vi "Teleop.vi"(10 "Match Info":T1={"Autonomous Elapsed Seconds"=0.0, "TeleOp Elapsed Seconds"=0.0, "Disabled Elapsed Seconds"=0.0, "Visited Autonomous"=FALSE, "Visited TeleOp"=FALSE, "Visited Disabled"=FALSE, "Autonomous Settings"={"Autonomous Style"=enum."Independent", "VI Refnum"=refnum}}, 11 "Call Context":T2) -> ()   [LabVIEW 2013]
doc: "This VI is called for each TeleOp packet received from the DS where the robot is not disabled. It is often used to read from the joysticks and update I/O or to update setpoints for timed control loops. It should complete and return within 20 milliseconds or it may miss DS packets."
uses:
  <vilib>/Rock Robotics/WPI/DriverStation/WPI_DriverStationDerivedRobotMode.ctl
  <vilib>/Rock Robotics/WPI/DriverStation/WPI_DriverStationMatch Info.ctl
  <vilib>/Rock Robotics/WPI/Solenoid/WPI_SolenoidValue.ctl
  <vilib>/Rock Robotics/WPI/Ultrasonic/WPI_UltrasonicRangeUnits.ctl
  Robot Global Data.vi
  <vilib>/Rock Robotics/WPI/Solenoid/WPI_SolenoidGetEnum.vi
  <vilib>/Rock Robotics/Network Tables/SD Read Number.vi
  <vilib>/Rock Robotics/WPI/Joystick/WPI_JoystickGetSetRefNum.vi
  <vilib>/Rock Robotics/WPI/Solenoid/WPI_SolenoidSetEnum.vi
  <vilib>/Rock Robotics/WPI/RobotDrive/WPI_RobotDriveGetSetRefNum.vi
panel:
  out "Waveform Chart":dbl(graph)
  in  "Fish Tester":dbl
  out "Sensor Time":dbl
  out "Ultrasonic Distance":dbl
  out "Mechanism Moving Up":bool
  out "Mechanism Moving Down":bool
  out "Time Since Button Pressed":dbl
  in  "Manual Override Activated":bool
  in  "Button 8 Pressed":bool
  out "Button 3":bool
  out "Button 2":bool
  out "Button 1":bool
  in  "Button 3 Pressed":bool
  in  "Button 2 Pressed":bool
  in  "Firing Pin Forward":bool
  in  "Mechanism Piston Forward":bool
  in  "Tick Taken":bool
  out "Time at Gather":dbl
  out "Time After Firing":dbl
  in  "Mechanism Status":string
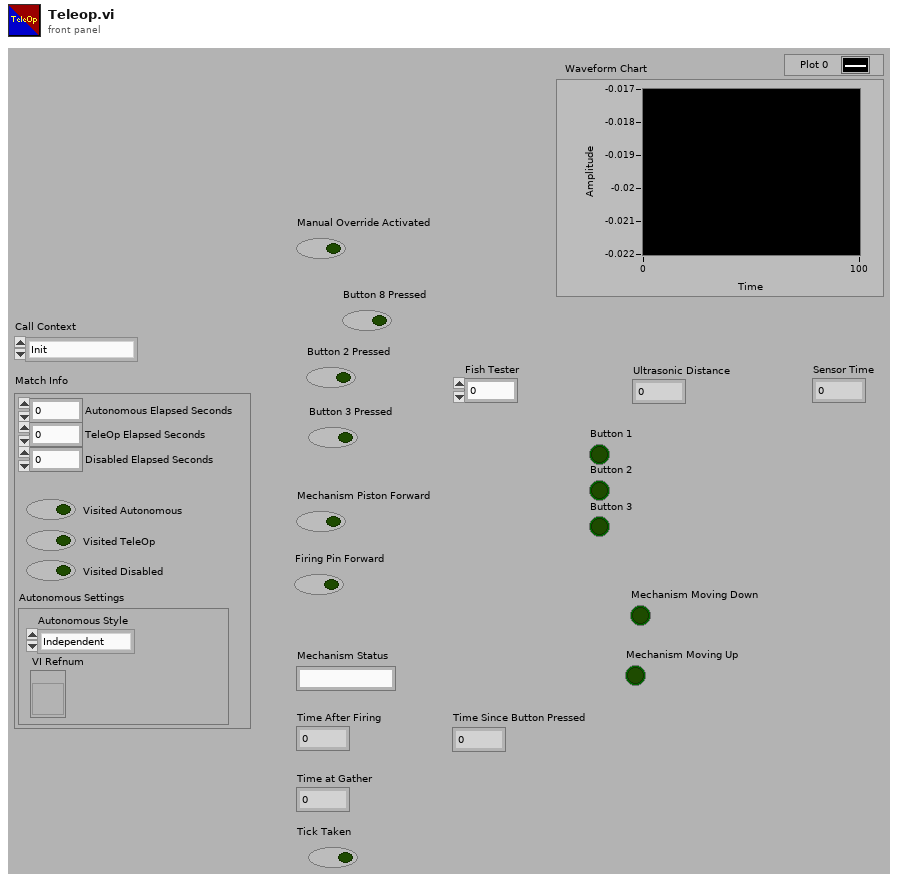
[diagram p1: front panel]
types:
  T1 = typedef "WPI_DriverStationMatch Info.ctl" = cluster{"Autonomous Elapsed Seconds":dbl, "TeleOp Elapsed Seconds":dbl, "Disabled Elapsed Seconds":dbl, "Visited Autonomous":bool, "Visited TeleOp":bool, "Visited Disabled":bool, "Autonomous Settings":cluster{"Autonomous Style":enum16{"Iterative", "Independent"}, "VI Refnum":refnum<vi>}}
  T2 = typedef "WPI_DriverStationDerivedRobotMode.ctl" = enum16{"Init", "Execute", "Stop"}
  T3 = typedef "WPI_SolenoidValue.ctl" = enum16{"Off", "On", "Forward", "Reverse"}
  T4 = typedef "WPI_JoystickDevRef.ctl" = cluster{"Device":T5}
  T5 = typedef "WPI_JoystickDeviceEnum.ctl" = enum16{"USB 1", "USB 2", "USB 3", "USB 4", "Kinect 1", "Kinect 2"}
  T6 = typedef "WPI_JoystickButtonState.ctl" = cluster{"Button 1":bool, "Button 2":bool, "Button 3":bool, "Button 4":bool, "Button 5":bool, "Button 6":bool, "Button 7":bool, "Button 8":bool, "Button 9":bool, "Button 10":bool, "Button 11":bool, "Button 12":bool}
  T7 = cluster{"axis 1 (x)":dbl, "axis 2 (y)":dbl, "axis 3 (throttle)":dbl, "axis 4":dbl, "axis 5":dbl, "axis 6":dbl}
  T8 = typedef "WPI_RobotDriveDevRef.ctl" = cluster{"DevStatus":errorcluster, "Motors[]":T9[], "Square Inputs":bool, "Max Output":dbl, "Isochronous":bool}
  T9 = typedef "WPI_MotorControlDeviceRef.ctl" = cluster{"DeviceStatus":errorcluster, "Type":enum16{"PWM", "CAN"}, "PWM":cluster{"Digital Module":T10, "PWM Channel":T11, "DeadBand":T12}, "CAN":cluster{"Device Number":u8, "Control Mode":T13, "Semaphore":T14, "Max Vout":dbl}, "Invert":bool, "TransformRef":T15, "InvTransformRef":T15}
  T10 = typedef "FPGA_TypedefDigitalModule.ctl" = enum16{"Digital Module 1", "Digital Module 2"}
  T11 = typedef "FPGA_DIOPWMChannel.ctl" = enum8{"PWM 1", "PWM 2", "PWM 3", "PWM 4", "PWM 5", "PWM 6", "PWM 7", "PWM 8", "PWM 9", "PWM 10", "Invalid"}
  T12 = typedef "WPI_PWMDeadband.ctl" = cluster{"Name":string, "maxPositivePwm":i32, "minPositivePwm":i32, "centerPwm":i32, "maxNegativePwm":i32, "minNegativePwm":i32, "angularRange":u16}
  T13 = typedef "WPI_CANJaguar_ControlMode.ctl" = enum8{"Percent VBus", "Current", "Speed", "Position", "Voltage"}
  T14 = typedef "Semaphore RefNum" = refnum<k1>
  T15 = typedef "WPI_PWMTransform_ConPane.ctl" = refnum<vi>
  T16 = typedef "WPI_SolenoidDevRef.ctl" = cluster{"DevStatus":errorcluster, "Solenoid Module":T17, "Forward Solenoid Channel":T18, "Reverse Solenoid Channel":T18}
  T17 = typedef "FPGA_TypedefSolenoidModule.ctl" = enum16{"Solenoid Module 1", "Solenoid Module 2"}
  T18 = typedef "WPI_SolenoidChannel.ctl" = enum8{"Solenoid 1", "Solenoid 2", "Solenoid 3", "Solenoid 4", "Solenoid 5", "Solenoid 6", "Solenoid 7", "Solenoid 8", "Invalid"}
  T19 = typedef "WPI_DigitalInputDevRef.ctl" = cluster{"DevStatus":errorcluster, "DIO Channel":T20, "Digital Module":T10}
  T20 = typedef "FPGA_DIOChannel.ctl" = enum8{"DIO 1", "DIO 2", "DIO 3", "DIO 4", "DIO 5", "DIO 6", "DIO 7", "DIO 8", "DIO 9", "DIO 10", "DIO 11", "DIO 12", "DIO 13", "DIO 14", "Invalid"}
  T21 = typedef "WPI_UltrasonicRangeUnits.ctl" = enum16{"inches", "mm"}
  T22 = typedef "WPI_UltrasonicDeviceRef.ctl" = cluster{"DevStatus":errorcluster, "Ping Digital Module":T10, "Echo Digital Module":T10, "Ping Channel":T20, "Echo Channel":T20, "CntIndex":T23}
  T23 = typedef "FPGA_CounterCtrSystemIndex.ctl" = enum8{"Ctr 0", "Ctr 1", "Ctr 2", "Ctr 3", "Ctr 4", "Ctr 5", "Ctr 6", "Ctr 7", "Invalid"}
  T24 = typedef "WPI_ServoDeviceRef.ctl" = cluster{"DeviceStatus":errorcluster, "Digital Module":T10, "PWM Channel":T11, "DeadBand":T12}
  T25 = typedef "WPI_AnalogChannelDevRef.ctl" = cluster{"DevStatus":errorcluster, "Analog Module":T26, "Analog Channel":T27}
  T26 = typedef "FPGA_TypedefAnalogModule.ctl" = enum16{"Analog Module 1", "Analog Module 2"}
  T27 = typedef "FPGA_AIChannel.ctl" = enum8{"AI 1", "AI 2", "AI 3", "AI 4", "AI 5", "AI 6", "AI 7", "AI 8", "Invalid"}
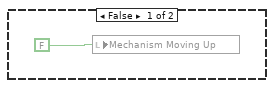
[diagram p2: hidden frame]
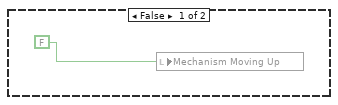
[diagram p3: hidden frame]
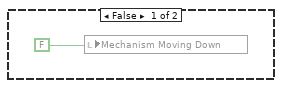
[diagram p4: hidden frame]
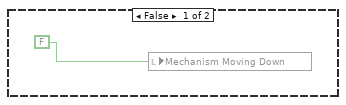
[diagram p5: hidden frame]
diagram:
  (unwired) "This code sets the toggle rate used by the Periodic Tasks VI.  For teleop mode we flash the USER1 LED on the cRIO at a fast rate.  Look at the Periodic Tasks VI to see how this global value is used."
  (unwired) "This VI is called each time a TeleOp DS packet is received.  Use it to respond to new joystick or Driver Station values.\n\nCommon tasks include reading the joysticks and updating motors, and updating setpoints for periodic loops.\n\nYou can open I/O on the FIRST Call, or in the Begin.vi."
  # "If no buttons pressed - 0\nIf left pressed = 7\nIf right pressed = -7\nIf both = 0"
  # "These are examples of reading dashboard variables."
  # "Publish the Robot Drive Motor\nvalues to the dashboard"
  # "Publish the joystick data the\nrobot sees to the dashboard"
  # "Each time we enter, report that\nwe are running teleop"
  # "Use to differentiate between\nFirst, Last, and Intermediate calls"
  # "This can help determine what has\nbeen run and for how long"
  # "Read Joystick X and Y values and update motor values"
  n1 = Unbundle By Name("Match Info") -> ()  [unwired: 1 out]
  n2 = local read "Time After Firing"() -> (w69:dbl)
  n3 = local read "Mechanism Status"() -> (w74:string)
  n4 = local write "Mechanism Piston Forward"(FALSE) -> ()
  n5 = local write "Firing Pin Forward"(FALSE) -> ()
  n6 = call <vilib>:"WPI_DriverStationReport Robot Code State.vi"("TeleOp"=TRUE ("Autonomous")) -> ()  [unwired: 10 in, 1 out]
  n7 = global write "Robot Global Data.vi" "LED toggle rate (ms)"(u32 100 ("LED ms toggle rate")) -> ()
  n8 = local read "Mechanism Status"() -> (w71:string)
  n9 = call <vilib>:"WPI_JoystickRefNum Registry Get.vi"("refnum name"="Joystick 1") -> ("JoystickDevRef"=w58:T4)  [unwired: 1 in, 9 out]
  n10 = call <vilib>:"WPI_JoystickRefNum Registry Get.vi"("refnum name"="Joystick 1") -> ("JoystickDevRef"=w76:T4)  [unwired: 1 in, 9 out]
  n11 = call <vilib>:"WPI_JoystickGet.vi"("JoystickDevRef"=w58) -> ("Buttons"=w57:T6)  [unwired: 1 in, 5 out]
  n12 = call <vilib>:"WPI_JoystickGet.vi"("JoystickDevRef"=w76) -> ("Buttons"=w75:T6, "Axes"=w55:T7)  [unwired: 1 in, 4 out]
  n13 = Tick Count (ms)() -> (millisecond timer value=w66:u32)
  n14 = call <vilib>:"WPI_RobotDriveRefNum Registry Get.vi"("refnum name"="Left and Right Motors") -> ("RobotDriveDevRef"=w90:T8)  [unwired: 1 in, 9 out]
  n15 = Unbundle By Name(w57) -> ("Button 8"=w56:bool)
  n16 = Unbundle By Name(w55) -> ()  [unwired: 1 out]
  n17 = call <vilib>:"WPI_SolenoidRefNum Registry Get.vi"("refnum name"="Firing Pin Solenoid") -> ("SolenoidDevRef"=w38:T16)  [unwired: 9 in, 1 out]
  n18 = call <vilib>:"SD Read Boolean.vi"("Name"="Manual Mechanism Override") -> ("Boolean"=w41:bool)  [unwired: 8 in, 2 out]
  n19 = call <vilib>:"WPI_SolenoidRefNum Registry Get.vi"("refnum name"="Mechanism Solenoid") -> ("SolenoidDevRef"=w32:T16)  [unwired: 9 in, 1 out]
  n20 = Subtract(x=w66, y=w69) -> (x-y=w68:dbl)
  n21 = Equal?(x=w74, y="Firing") -> (x = y?=w72:bool)
  n22 = case shown="True" w72 {
    frame False {
    }
    frame True {
      n23 = Tick Count (ms)() -> (millisecond timer value=w94:u32)
      n24 = local write "Firing Pin Forward"(FALSE) -> ()
      n25 = local write "Time After Firing"(w94) -> ()
      n26 = local write "Mechanism Status"("Resetting") -> ()
      n27 = call <vilib>:"WPI_SolenoidRefNum Registry Get.vi"("refnum name"="Firing Pin Solenoid") -> ("SolenoidDevRef"=w97:T16)  [unwired: 9 in, 1 out]
      n28 = call-poly <vilib>:"WPI_SolenoidSet.vi"("Value"=WPI_SolenoidValue."Reverse", "SolenoidDevRef"=w97) -> ()  [unwired: 8 in, 2 out]
    }
  }
  n29 = case shown="True" w41 {
    tunnel: w38 -> [_ w114]
    tunnel: w32 -> [_ w113]
    frame False {
    }
    frame True {
      n30 = call <vilib>:"SD Read Boolean.vi"("Name"="Firing Pin Piston Extended") -> ("Boolean"=w104:bool)  [unwired: 8 in, 2 out]
      n31 = call <vilib>:"SD Read Boolean.vi"("Name"="Mechanism Piston Extended") -> ("Boolean"=w111:bool)  [unwired: 8 in, 2 out]
      n32 = Equal?(x=w104, y=TRUE) -> (x = y?=w102:bool)
      n33 = Equal?(x=w111, y=TRUE) -> (x = y?=w109:bool)
      n34 = Select(t=WPI_SolenoidValue."Forward" ("Value"), s=w102, f=WPI_SolenoidValue."Reverse") -> (s? t:f=w99:T3)
      n35 = Select(t=WPI_SolenoidValue."Forward" ("Value"), s=w109, f=WPI_SolenoidValue."Reverse") -> (s? t:f=w106:T3)
      n36 = call-poly <vilib>:"WPI_SolenoidSet.vi"("Value"=w99, "SolenoidDevRef"=w114) -> ()  [unwired: 8 in, 2 out]
      n37 = call-poly <vilib>:"WPI_SolenoidSet.vi"("Value"=w106, "SolenoidDevRef"=w113) -> ()  [unwired: 8 in, 2 out]
    }
  }
  n38 = Unbundle By Name(w75) -> ("Button 1"=w60:bool, "Button 2"=w28:bool, "Button 3"=w27:bool, "Button 5"=w46:bool, "Button 6"=w47:bool)
  "Button 1" <- w60
  "Button 3" <- w27
  "Button 2" <- w28
  n39 = disable-structure shown="Disabled" {
    disable-tunnel: w28 -> [w116 _]
    disable-tunnel: w27 -> [w115 _]
    frame Disabled {
      n40 = case shown="True" w116 {
        frame False {
          n41 = local write "Mechanism Moving Down"(FALSE) -> ()
        }
        frame True {
          n42 = call <vilib>:"WPI_DigitalInputRefNum Registry Get.vi"("refnum name"="Bottom Limit Switch") -> ("DigitalInputDevRef"=w129:T19)  [unwired: 9 in, 1 out]
          n43 = call <vilib>:"WPI_DigitalInputGetValue.vi"("DigitalInputDevRef"=w129) -> ("Value"=w127:bool)  [unwired: 8 in, 2 out]
          n44 = case shown="True" w127 {
            frame False {
              n45 = local write "Mechanism Moving Down"(FALSE) -> ()
            }
            frame True {
              n46 = call <vilib>:"WPI_MotorControlRefNum Registry Get.vi"("refnum name"="Mechanism Motor 1") -> ("MotorControlDevRef"=w133:T9)  [unwired: 9 in, 1 out]
              n47 = call <vilib>:"WPI_MotorControlSetOutput.vi"("Output"=-0.1, "MotorControlDevRef"=w133) -> ()  [unwired: 7 in, 3 out]
              n48 = local write "Mechanism Moving Down"(TRUE) -> ()
            }
          }
        }
      }
      n49 = case shown="True" w115 {
        frame False {
          n50 = local write "Mechanism Moving Up"(FALSE) -> ()
        }
        frame True {
          n51 = call <vilib>:"WPI_DigitalInputRefNum Registry Get.vi"("refnum name"="Top Limit Switch") -> ("DigitalInputDevRef"=w120:T19)  [unwired: 9 in, 1 out]
          n52 = call <vilib>:"WPI_DigitalInputGetValue.vi"("DigitalInputDevRef"=w120) -> ("Value"=w118:bool)  [unwired: 8 in, 2 out]
          n53 = case shown="True" w118 {
            frame False {
              n54 = local write "Mechanism Moving Up"(FALSE) -> ()
            }
            frame True {
              n55 = call <vilib>:"WPI_MotorControlRefNum Registry Get.vi"("refnum name"="Mechanism Motor 1") -> ("MotorControlDevRef"=w124:T9)  [unwired: 9 in, 1 out]
              n56 = call <vilib>:"WPI_MotorControlSetOutput.vi"("Output"=0.1, "MotorControlDevRef"=w124) -> ()  [unwired: 7 in, 3 out]
              n57 = local write "Mechanism Moving Up"(TRUE) -> ()
            }
          }
        }
      }
    }
    frame Enabled {
    }
  }
  n58 = call-poly <vilib>:"WPI_SolenoidGet.vi"("SolenoidDevRef"=w38) -> ("Value"=w36:T3)  [unwired: 8 in, 2 out]
  n59 = call-poly <vilib>:"WPI_SolenoidGet.vi"("SolenoidDevRef"=w32) -> ("Value"=w31:T3)  [unwired: 8 in, 2 out]
  n60 = case shown="True" w56 {
    frame False {
    }
    frame True {
      n61 = global read "Robot Global Data.vi" "Time since  button 8 pressed"() -> (w135:dbl)
      n62 = Tick Count (ms)() -> (millisecond timer value=w139:u32)
      n63 = Subtract(x=w139, y=w135) -> (x-y=w138:dbl)
      n64 = Greater?(x=w138, y=300) -> (0:w136:bool)
      n65 = case shown="True" w136 {
        frame False {
        }
        frame True {
          n66 = Tick Count (ms)() -> (millisecond timer value=w140:u32)
          n67 = local read "Manual Override Activated"() -> (w144:bool)
          n68 = global write "Robot Global Data.vi" "Time since  button 8 pressed"(w140) -> ()
          n69 = Select(t=FALSE, s=w144, f=TRUE) -> (s? t:f=w141:bool)
          n70 = local write "Manual Override Activated"(w141) -> ()
        }
      }
    }
  }
  n71 = Equal?(x=w71, y="Resetting") -> (x = y?=w65:bool)
  n72 = Equal?(x=w36, y=WPI_SolenoidValue."Forward") -> (x = y?=w34:bool)
  n73 = Equal?(x=w31, y=WPI_SolenoidValue."Forward") -> (x = y?=w30:bool)
  n74 = Greater Or Equal?(x=3000, y=w68) -> (x >= y?=w64:bool)
  n75 = And(x=w65, y=w64) -> (x .and. y?=w63:bool)
  n76 = call <vilib>:"SD Write Boolean.vi"("Boolean"=w34, "Name"="Is The Firing Pin Piston Extended") -> ()  [unwired: 8 in, 2 out]
  n77 = call <vilib>:"SD Write Boolean.vi"("Boolean"=w30, "Name"="Are Mechanism Pistons Extended") -> ()  [unwired: 8 in, 2 out]
  n78 = call <vilib>:"WPI_JoystickRefNum Registry Get.vi"("refnum name"="Joystick 1") -> ("JoystickDevRef"=w88:T4)  [unwired: 1 in, 9 out]
  n79 = case shown="True" w63 {
    frame False {
    }
    frame True {
      n80 = call <vilib>:"WPI_DigitalInputRefNum Registry Get.vi"("refnum name"="Micro Switch 1") -> ("error out"=w155:errorcluster, "DigitalInputDevRef"=w154:T19)  [unwired: 9 in]
      n81 = call <vilib>:"WPI_DigitalInputRefNum Registry Get.vi"("refnum name"="Reed Switch 1") -> ("DigitalInputDevRef"=w146:T19)  [unwired: 9 in, 1 out]
      n82 = call <vilib>:"WPI_SolenoidRefNum Registry Get.vi"("refnum name"="Firing Pin Solenoid") -> ("SolenoidDevRef"=w147:T16)  [unwired: 9 in, 1 out]
      n83 = call <vilib>:"WPI_DigitalInputRefNum Registry Get.vi"("refnum name"="Reed Switch 2") -> ("DigitalInputDevRef"=w145:T19)  [unwired: 9 in, 1 out]
      n84 = call <vilib>:"WPI_SolenoidRefNum Registry Get.vi"("refnum name"="Mechanism Solenoid") -> ("SolenoidDevRef"=w150:T16)  [unwired: 9 in, 1 out]
      n85 = call <vilib>:"WPI_DigitalInputGetValue.vi"("error in (no error)"=w155, "DigitalInputDevRef"=w154) -> ("Value"=w151:bool)  [unwired: 7 in, 2 out]
      n86 = case shown="True" w151 {
        tunnel: w146 -> [_ w169]
        tunnel: w150 -> [w158 w167]
        tunnel: w147 -> [w159 _]
        tunnel: w145 -> [w157 _]
        frame False {
          n87 = call <vilib>:"WPI_DigitalInputGetValue.vi"("DigitalInputDevRef"=w157) -> ("Value"=w160:bool)  [unwired: 8 in, 2 out]
          n88 = case shown="False" w160 {
            tunnel: w159 -> [_ w166]
            tunnel: w158 -> [w163 _]
            frame False {
              n89 = local write "Mechanism Piston Forward"(TRUE) -> ()
              n90 = call-poly <vilib>:"WPI_SolenoidSet.vi"("Value"=WPI_SolenoidValue."Forward", "SolenoidDevRef"=w163) -> ()  [unwired: 8 in, 2 out]
            }
            frame True {
              n91 = local write "Firing Pin Forward"(TRUE) -> ()
              n92 = call-poly <vilib>:"WPI_SolenoidSet.vi"("Value"=WPI_SolenoidValue."Forward", "SolenoidDevRef"=w166) -> ()  [unwired: 8 in, 2 out]
            }
          }
        }
        frame True {
          n93 = call <vilib>:"WPI_DigitalInputGetValue.vi"("DigitalInputDevRef"=w169) -> ("Value"=w168:bool)  [unwired: 8 in, 2 out]
          n94 = case shown="True" w168 {
            tunnel: w167 -> [w172 _]
            frame False {
              n95 = local write "Mechanism Piston Forward"(FALSE) -> ()
              n96 = call-poly <vilib>:"WPI_SolenoidSet.vi"("Value"=WPI_SolenoidValue."Reverse", "SolenoidDevRef"=w172) -> ()  [unwired: 8 in, 2 out]
            }
            frame True {
              n97 = local write "Mechanism Status"("Ready To Fire") -> ()
            }
          }
        }
      }
    }
  }
  n98 = case shown="True" w60 {
    frame False {
    }
    frame True {
      n99 = local read "Mechanism Status"() -> (w175:string)
      n100 = Equal?(x=w175, y="Ready To Fire") -> (x = y?=w174:bool)
      n101 = case shown="True" w174 {
        frame False {
        }
        frame True {
          n102 = local write "Mechanism Status"("Firing") -> ()
        }
      }
    }
  }
  n103 = And(x=w47, y=w46) -> (x .and. y?=w48:bool)
  n104 = call <vilib>:"WPI_JoystickGet.vi"("JoystickDevRef"=w88) -> ("Buttons"=w86:T6, "Axes"=w83:T7)  [unwired: 1 in, 4 out]
  n105 = local read "Mechanism Moving Down"() -> (w24:bool)
  n106 = call <vilib>:"WPI_JoystickRefNum Registry Get.vi"("refnum name"="Joystick 1") -> ("JoystickDevRef"=w12:T4)  [unwired: 1 in, 9 out]
  n107 = local read "Mechanism Moving Up"() -> (w25:bool)
  n108 = Select(t=7.0, s=w46, f=0.0) -> (s? t:f=w49:dbl)
  n109 = Cluster To Array(cluster=w86) -> (array=w85:bool[])
  n110 = call <vilib>:"WPI_JoystickGet.vi"("JoystickDevRef"=w12) -> ("Buttons"=w11:T6)  [unwired: 1 in, 5 out]
  n111 = Cluster To Array(cluster=w83) -> (array=w82:dbl[])
  n112 = Unbundle By Name(w83) -> ("axis 1 (x)"=w5:dbl, "axis 2 (y)"=w3:dbl, "axis 3 (throttle)"=w1:dbl)
  n113 = disable-structure shown="Enabled" {
    disable-tunnel: w1 -> [_ w179]
    frame Disabled {
    }
    frame Enabled {
      n114 = call <vilib>:"WPI_MotorControlRefNum Registry Get.vi"("refnum name"="Mechanism Motor 1") -> ("error out"=w178:errorcluster, "MotorControlDevRef"=w180:T9)  [unwired: 9 in]
      n115 = call <vilib>:"WPI_MotorControlSetOutput.vi"("error in (no error)"=w178, "Output"=w179, "MotorControlDevRef"=w180) -> ()  [unwired: 6 in, 3 out]
    }
  }
  n116 = Select(t=-7.0, s=w47, f=w49) -> (s? t:f=w45:dbl)
  n117 = Unbundle By Name(w11) -> ("Button 4"=w10:bool)
  n118 = Negate(x=w5) -> (-x=w4:dbl)
  n119 = call <vilib>:"WPI_MotorControlRefNum Registry Get.vi"("refnum name"="Mechanism Motor 2") -> ("MotorControlDevRef"=w50:T9)  [unwired: 9 in, 1 out]
  n120 = call <vilib>:"SD Write Numeric Array.vi"("Numeric Array"=w82, "Name"="Joystick 1/Axes") -> ()  [unwired: 8 in, 2 out]
  n121 = Select(t=w45, s=w48, f=0.0) -> (s? t:f=w43:dbl)
  n122 = call <vilib>:"WPI_SolenoidRefNum Registry Get.vi"("refnum name"="Grabber Pistons Solenoid") -> ("SolenoidDevRef"=w8:T16)  [unwired: 9 in, 1 out]
  n123 = Not(x=w25) -> (.not. x?=w23:bool)
  n124 = Not(x=w24) -> (.not. x?=w22:bool)
  n125 = Negate(x=w3) -> (-x=w2:dbl)
  n126 = call <vilib>:"WPI_RobotDriveArcadeDrive_Standard(NoSaturation).vi"("Y axis value"=w2, "X axis value"=w4, "RobotDriveDevRef"=w90) -> ("Motor Values"=w79:dbl[])  [unwired: 1 in, 7 out]
  n127 = call <vilib>:"SD Write Numeric Array.vi"("Numeric Array"=w79, "Name"="RobotDrive Motors") -> ()  [unwired: 8 in, 2 out]
  n128 = call <vilib>:"WPI_MotorControlSetOutput.vi"("Output"=w43, "MotorControlDevRef"=w50) -> ()  [unwired: 7 in, 3 out]
  n129 = And(x=w23, y=w22) -> (x .and. y?=w26:bool)
  n130 = case shown="True" w10 {
    tunnel: w8 -> [_ w192]
    frame False {
    }
    frame True {
      n131 = call-poly <vilib>:"WPI_SolenoidSet.vi"("Value"=WPI_SolenoidValue."Reverse", "SolenoidDevRef"=w192) -> ()  [unwired: 8 in, 2 out]
      n132 = call <vilib>:"WPI_MotorControlRefNum Registry Get.vi"("refnum name"="Mechanism Motor 2") -> ("MotorControlDevRef"=w189:T9)  [unwired: 9 in, 1 out]
      n133 = call <vilib>:"WPI_MotorControlSetOutput.vi"("Output"=-7.0, "MotorControlDevRef"=w189) -> ()  [unwired: 7 in, 3 out]
      n134 = call <vilib>:"WPI_UltrasonicRefNum Registry Get.vi"("refnum name"="Grabber Ultrasonic Sensor") -> ("UltrasonicDevRef"=w186:T22)  [unwired: 9 in, 1 out]
      n135 = call <vilib>:"WPI_UltrasonicGetRange.vi"("Range Units"=WPI_UltrasonicRangeUnits."inches", "UltrasonicDevRef"=w186) -> ("Distance"=w184:dbl)  [unwired: 7 in, 2 out]
      n136 = Less?(x=w184, y=6.0) -> (x < y?=w182:bool)
      n137 = case shown="True" w182 {
        frame False {
        }
        frame True {
          n138 = call <vilib>:"WPI_DigitalInputRefNum Registry Get.vi"("refnum name"="Top Limit  Switch") -> ("DigitalInputDevRef"=w194:T19)  [unwired: 9 in, 1 out]
          n139 = call <vilib>:"WPI_DigitalInputGetValue.vi"("DigitalInputDevRef"=w194) -> ("Value"=w193:bool)  [unwired: 8 in, 2 out]
          n140 = case shown="False" w193 {
            frame False {
            }
            frame True {
            }
          }
        }
      }
    }
  }
  n141 = case shown="True" w26 {
    frame False {
    }
    frame True {
      n142 = call <vilib>:"WPI_MotorControlRefNum Registry Get.vi"("refnum name"="Mechanism Motor 1") -> ("MotorControlDevRef"=w198:T9)  [unwired: 9 in, 1 out]
      n143 = call <vilib>:"WPI_MotorControlSetOutput.vi"("Output"=0.0, "MotorControlDevRef"=w198) -> ()  [unwired: 7 in, 3 out]
    }
  }
  n144 = call <vilib>:"SD Write Boolean Array.vi"("Boolean Array"=w85, "Name"="Joystick 1/Buttons") -> ()  [unwired: 8 in, 2 out]
  n145 = call-poly <vilib>:"SD Read Value.vi"("Name"="Camera Pitch Control") -> ("Numeric"=w14:dbl)  [unwired: 8 in, 2 out]
  n146 = call <vilib>:"WPI_ServoRefNum Registry Get.vi"("refnum name"="Camera Pitch Servo") -> ("ServoDeviceRef"=w15:T24)  [unwired: 9 in, 1 out]
  n147 = call-poly <vilib>:"SD Read Value.vi"("Name"="Camera Rotation Control") -> ("Numeric"=w18:dbl)  [unwired: 8 in, 2 out]
  n148 = call <vilib>:"WPI_ServoRefNum Registry Get.vi"("refnum name"="Camera Rotation Servo") -> ("ServoDeviceRef"=w17:T24)  [unwired: 9 in, 1 out]
  n149 = call <vilib>:"WPI_ServoSetPosition.vi"("Position"=w14, "ServoDeviceRef"=w15) -> ()  [unwired: 8 in, 2 out]
  n150 = call <vilib>:"WPI_ServoSetPosition.vi"("Position"=w18, "ServoDeviceRef"=w17) -> ()  [unwired: 8 in, 2 out]
  n151 = disable-structure shown="Disabled" {
    frame Disabled {
      n152 = call <vilib>:"WPI_DigitalInputRefNum Registry Get.vi"("refnum name"="Top Limit Switch") -> ("DigitalInputDevRef"=w202:T19)  [unwired: 9 in, 1 out]
      n153 = call <vilib>:"WPI_DigitalInputGetValue.vi"("DigitalInputDevRef"=w202) -> ("Value"=w200:bool)  [unwired: 8 in, 2 out]
      n154 = Not(x=w200) -> (.not. x?=w199:bool)
      n155 = And(x=w199) -> (x .and. y?=w201:bool)  [unwired: 1 in]
      n156 = case shown="True" w201 {
        frame False {
        }
        frame True {
          n157 = call <vilib>:"WPI_MotorControlRefNum Registry Get.vi"("refnum name"="Mechanism Motor 1") -> ("MotorControlDevRef"=w206:T9)  [unwired: 9 in, 1 out]
          n158 = call <vilib>:"WPI_MotorControlSetOutput.vi"("Output"=0.5, "MotorControlDevRef"=w206) -> ()  [unwired: 7 in, 3 out]
        }
      }
    }
    frame Enabled {
    }
  }
  n159 = disable-structure shown="Disabled" {
    frame Disabled {
      n160 = call <vilib>:"WPI_DigitalInputRefNum Registry Get.vi"("refnum name"="Bottom Limit Switch") -> ("DigitalInputDevRef"=w208:T19)  [unwired: 9 in, 1 out]
      n161 = call <vilib>:"WPI_DigitalInputGetValue.vi"("DigitalInputDevRef"=w208) -> ("Value"=w210:bool)  [unwired: 8 in, 2 out]
      n162 = Not(x=w210) -> (.not. x?=w209:bool)
      n163 = And(x=w209) -> (x .and. y?=w207:bool)  [unwired: 1 in]
      n164 = case shown="True" w207 {
        frame False {
        }
        frame True {
          n165 = call <vilib>:"WPI_MotorControlRefNum Registry Get.vi"("refnum name"="Mechanism Motor 1") -> ("MotorControlDevRef"=w214:T9)  [unwired: 9 in, 1 out]
          n166 = call <vilib>:"WPI_MotorControlSetOutput.vi"("Output"=-0.5, "MotorControlDevRef"=w214) -> ()  [unwired: 7 in, 3 out]
        }
      }
    }
    frame Enabled {
    }
  }
  n167 = flat-sequence {
    tunnel: [w215] -> w6
    tunnel: [w219] -> w7
    tunnel: w6 -> [w219]
    tunnel: w7 -> [w220]
    frame #0 {
      n168 = Tick Count (ms)() -> (millisecond timer value=w215:u32)
    }
    frame #1 {
      n169 = call <vilib>:"WPI_AnalogChannelRefNum Registry Get.vi"("refnum name"="Grabber Ultrasonic Sensor") -> ("AIDeviceRef"=w217:T25)  [unwired: 9 in, 1 out]
      n170 = call <vilib>:"WPI_AnalogChannelGetAverageVoltage.vi"("AIDeviceRef"=w217) -> ("Voltage"=→"Ultrasonic Distance" →"Waveform Chart":dbl)  [unwired: 8 in, 2 out]
    }
    frame #2 {
      n171 = Tick Count (ms)() -> (millisecond timer value=w221:u32)
      n172 = Subtract(x=w221, y=w220) -> (x-y=→"Sensor Time":u32)
    }
  }
  n173 = disable-structure shown="Disabled" {
    frame Disabled {
      n174 = call <vilib>:"WPI_MotorControlRefNum Registry Get.vi"("refnum name"="Fish Test") -> ("MotorControlDevRef"=w224:T9)  [unwired: 9 in, 1 out]
      n175 = call <vilib>:"WPI_MotorControlSetOutput.vi"("Output"="Fish Tester", "MotorControlDevRef"=w224) -> ()  [unwired: 7 in, 3 out]
    }
    frame Enabled {
    }
  }
